vi "Push_Multi_Unsat_Warp.vi"   [LabVIEW 2024, in "POTCircularBuffer.Tests.Units.lvlib"]
uses:
  POTCircularBuffer.Tests.Units.lvlib
  POTTypedCircularBuffer.lvclass
  Type.ctl
  <vilib>/addons/_JKI Toolkits/Caraya/classes/Test/Test.lvclass
  <vilib>/addons/_JKI Toolkits/Caraya/classes/Assert/Assert.lvclass
  <vilib>/addons/_JKI Toolkits/Caraya/classes/Assert/Assert Equal Value and Type_Variant.vi
types:
  T1 = typedef "POTTypedCircularBuffer.lvclass/Type.ctl" = i32
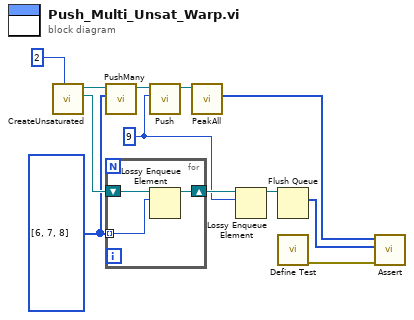
[diagram p0: block diagram]
diagram:
  w8 = T1[] [6, 7, 8] ("Elements")
  w6 = T1 9 ("Element")
  n1 = call "CreateUnsaturated.vi"("unsat amount (2)"=2) -> ("Golden"=w9:refnum<queue>, "POTTypedCircularBuffer out"=w10:refnum<class "POTTypedCircularBuffer.lvclass">)  [unwired: 9 in]
  n2 = call "PushMany.vi"("Elements"=w8, "POTTypedCircularBuffer in"=w10) -> ("POTTypedCircularBuffer out"=w11:refnum<class "POTTypedCircularBuffer.lvclass">)  [unwired: 9 in]
  n3 = for {
    tunnel: w8 -> [w14] mode=indexing
    shift-right: [w13] -> w7
    shift-left: w9 -> [w15]
    n4 = Lossy Enqueue Element(queue=w15, element=w14) -> (queue out=w13:refnum<queue>)  [unwired: 1 in, 3 out]
  }
  n5 = call "Push.vi"("Element"=w6, "POTTypedCircularBuffer in"=w11) -> ("POTTypedCircularBuffer out"=w12:refnum<class "POTTypedCircularBuffer.lvclass">)  [unwired: 9 in]
  n6 = call "PeakAll.vi"("POTTypedCircularBuffer in"=w12) -> ("Copied Buffer"=w2:T1[])  [unwired: 9 in, 1 out]
  n7 = Lossy Enqueue Element(queue=w7, element=w6) -> (queue out=w5:refnum<queue>)  [unwired: 1 in, 3 out]
  n8 = Flush Queue(queue=w5) -> (remaining elements=w1:T1[])  [unwired: 1 in, 2 out]
  n9 = call <vilib>:"Define Test.vi"() -> ("error out"=w4:errorcluster)  [unwired: 10 in, 1 out]
  n10 = call-poly <vilib>:"Assert.vi"("error in (no error)"=w4, "Y"=w1, "X"=w2) -> ()  [unwired: 7 in, 2 out]
